vi "Command Move Direction Field (Gyro Hold).vi"(2 "Input Robot System Funtions":T1, 3 "Cmd Parameter 1":dbl, 4 "Cmd Parameter 2":dbl, 5 "Startup":bool) -> (0 "Output Robot System Functions":T1, 1 "Completed":bool)   [LabVIEW 2014]
uses:
  Subsystems VIs/Robot Commands.ctl
  Command Execution State.ctl
  Global Variables/Sensor Data (Edited).vi
  Global Variables/Settings.vi
panel:
  out "PID Tracking":cluster{"Goal Wheel Position":dbl, dbl}(graph)={"Goal Wheel Position"=0.0, -90.17571233858979}
  # "Sample robot\ncontrol output.\nReplace with \nactual teleop \ncontrol signal \nstructure."
  # "Field Centric"
  # "Field Centric"
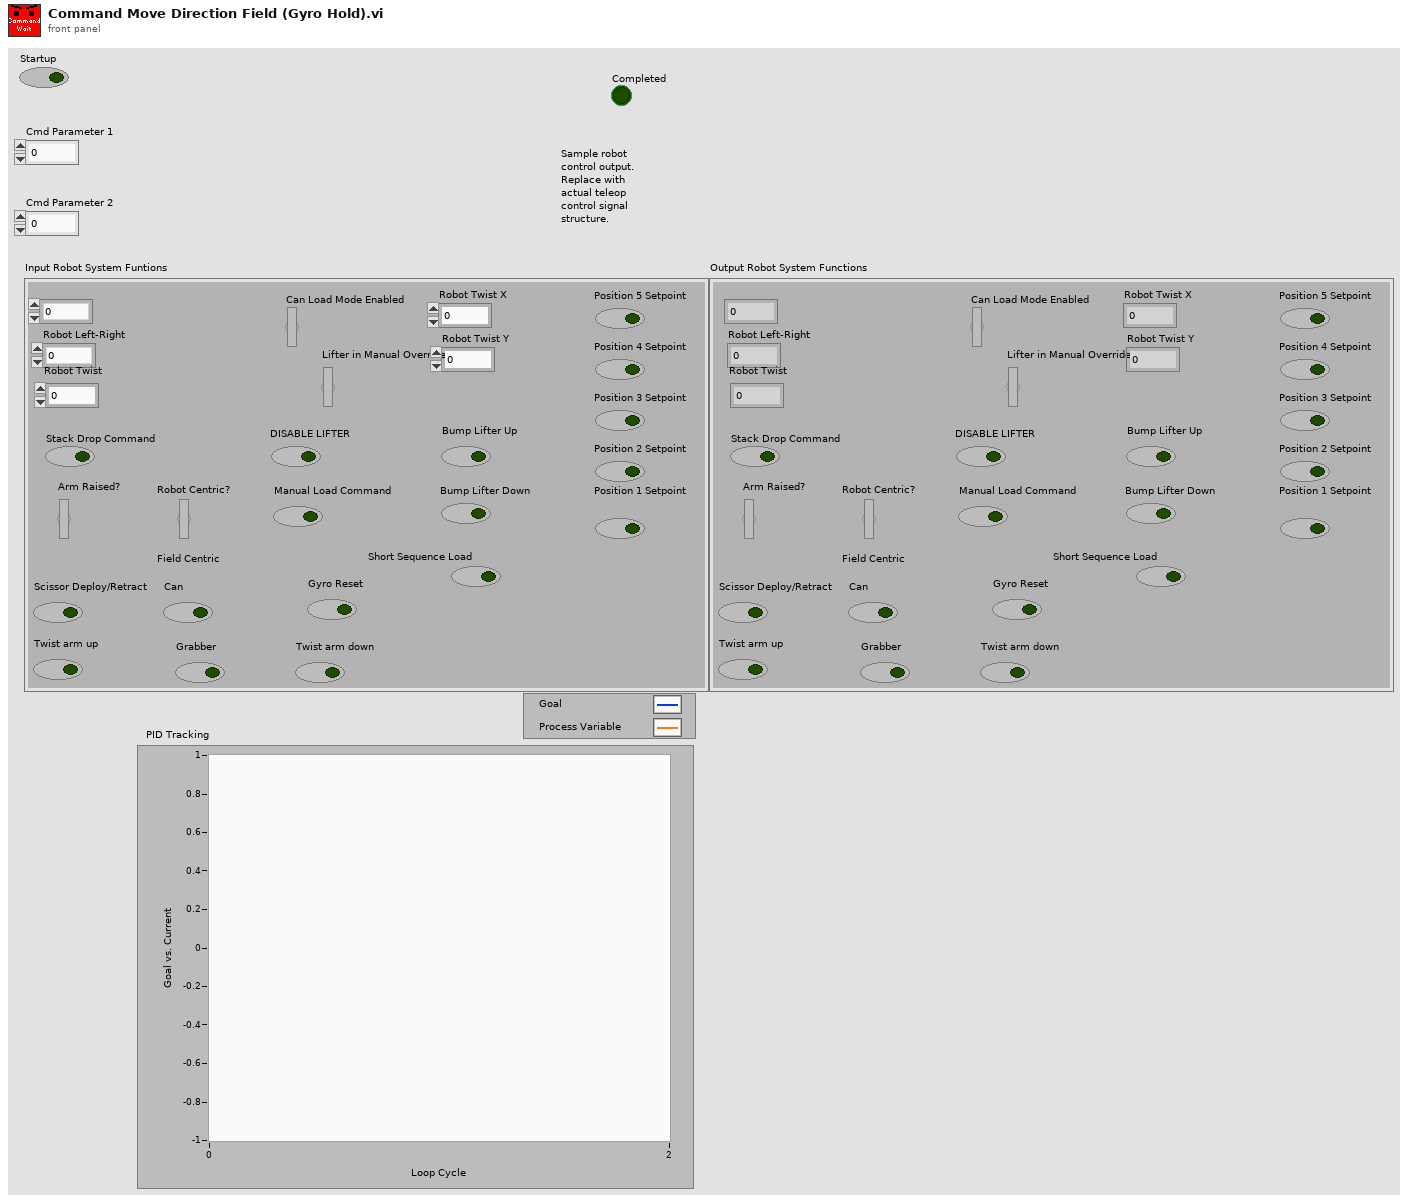
[diagram p1: front panel]
types:
  T1 = typedef "Robot Commands.ctl" = cluster{"Robot Forward-Reverse":dbl, "Robot Left-Right":dbl, "Robot Twist":dbl, "Can Load Mode Enabled":bool, "Lifter in Manual Override?":bool, "Stack Drop Command":bool, "Arm Raised?":bool, "DISABLE LIFTER":bool, "Position 1 Setpoint":bool, "Position 2 Setpoint":bool, "Position 3 Setpoint":bool, "Position 4 Setpoint":bool, "Position 5 Setpoint":bool, "Bump Lifter Down":bool, "Bump Lifter Up":bool, "Manual Load Command":bool, "Robot Centric?":bool, "Scissor Deploy/Retract":bool, "Grabber":bool, "Can":bool, "Twist arm up":bool, "Gyro Reset":bool, "Twist arm down":bool, "Short Sequence Load":bool, "Robot Twist X":dbl, "Robot Twist Y":dbl}
  T2 = typedef "Command Execution State.ctl" = enum16{"Initialize", "Execute", "Finish"}
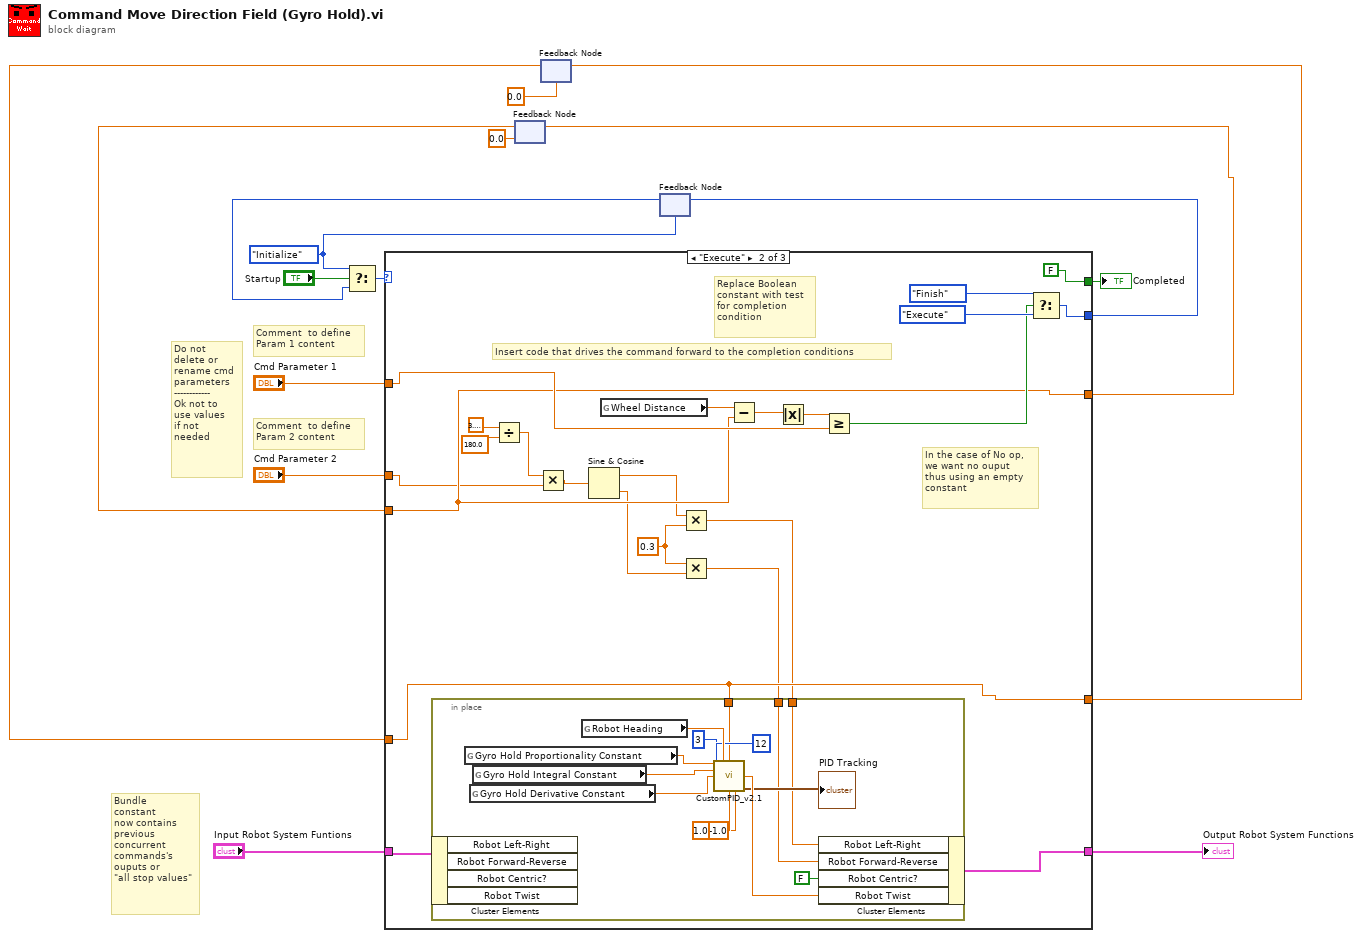
[diagram p0: block diagram]
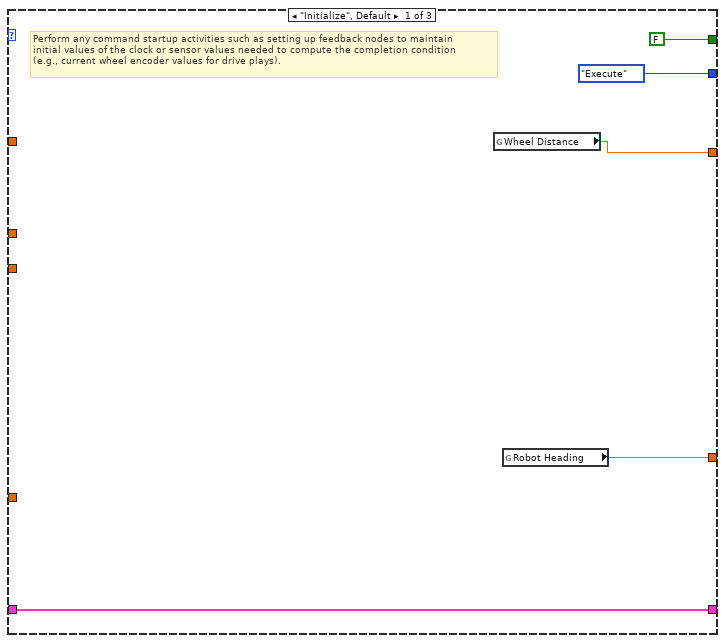
[diagram p2: hidden frame]
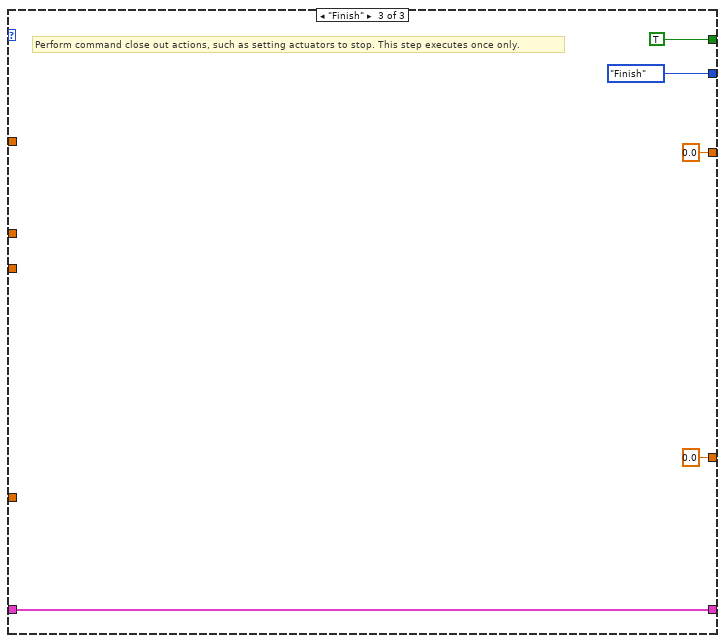
[diagram p3: hidden frame]
diagram:
  w11 = Command_Execution_State."Initialize" ("Play State")
  # "Bundle \nconstant\nnow contains\nprevious \nconcurrent\ncommands's\nouputs or\n\"all stop values\""
  # "Do not \ndelete or\nrename cmd\nparameters\n------------\nOk not to \nuse values\nif not \nneeded"
  # "Comment  to define\nParam 2 content"
  # "Comment  to define\nParam 1 content"
  n1 = feedback #1(0.0 ("Wheel Distance")) -> (w5:dbl)
  n2 = feedback #2(0.0 ("Wheel Distance")) -> (w2:dbl)
  n3 = feedback #3(w11) -> (w12:T2)
  n4 = Select(t=w11, s="Startup", f=w12) -> (s? t:f=w16:T2)
  n5 = case shown="\"Execute\"" w16 {
    tunnel: [FALSE FALSE TRUE] -> w14
    tunnel: [Command_Execution_State."Execute" ("Play State") w35 Command_Execution_State."Finish" ("f")] -> w13
    tunnel: "Cmd Parameter 1" -> [_ w36 _]
    tunnel: "Cmd Parameter 2" -> [_ w29 _]
    tunnel: [w19 w37 w59] -> w7
    tunnel: "Input Robot System Funtions" -> [w19 w38 w59]
    tunnel: [w18 w33 0.0 ("Wheel Distance")] -> w6
    tunnel: w5 -> [_ w33 _]
    tunnel: [w17 w28 0.0 ("Wheel Distance")] -> w3
    tunnel: w2 -> [_ w28 _]
    frame "Initialize", Default {
      # "Perform any command startup activities such as setting up feedback nodes to maintain \ninitial values of the clock or sensor values needed to compute the completion condition\n(e.g., current wheel encoder values for drive plays)."
      n6 = global read "Sensor Data (Edited).vi" "Wheel Distance"() -> (w18:dbl)
      n7 = global read "Sensor Data (Edited).vi" "Robot Heading"() -> (w17:dbl)
    }
    frame "Execute" {
      w24 = 0.3
      # "In the case of No op, \nwe want no ouput \nthus using an empty \nconstant"
      # "Replace Boolean\nconstant with test \nfor completion \ncondition"
      # "Insert code that drives the command forward to the completion conditions"
      n8 = Divide(x=3.141592653589793, y=180.0) -> (x/y=w30:dbl)
      n9 = Multiply(x=w30, y=w29) -> (x*y=w27:dbl)
      n10 = Sine & Cosine(0:w27) -> (1:w26:dbl, 2:w25:dbl)
      n11 = global read "Sensor Data (Edited).vi" "Wheel Distance"() -> (w44:dbl)
      n12 = Multiply(x=w26, y=w24) -> (x*y=w22:dbl)
      n13 = Multiply(x=w24, y=w25) -> (x*y=w23:dbl)
      n14 = in-place {
        in-place-border: w28 -> [w47]
        in-place-border: w23 -> [w45]
        in-place-border: w22 -> [w46]
        n15 = in-place-cluster #4(w38) -> ()  [unwired: 4 out]
        n16 = global read "Settings.vi" "Gyro Hold Proportionality Constant"() -> (w51:dbl)
        n17 = global read "Settings.vi" "Gyro Hold Derivative Constant"() -> (w49:dbl)
        n18 = global read "Settings.vi" "Gyro Hold Integral Constant"() -> (w50:dbl)
        n19 = global read "Sensor Data (Edited).vi" "Robot Heading"() -> (w56:dbl)
        n20 = call "CustomPID_v2.1.vi"("Kp"=w51, "Process Variable"=w56, "Goal"=w47, "Ki"=w50, "Kd"=w49, "N-Diff"=3, "N-Int"=12, "Max Ouput"=1.0, "Min Output"=-1.0) -> ("Command"=w57:dbl, "PID Tracking"=→"PID Tracking":cluster{"Goal Wheel Position":dbl, dbl})  [unwired: 4 in, 1 out]
        n21 = in-place-cluster #4("Robot Left-Right"=w46, "Robot Forward-Reverse"=w45, "Robot Centric?"=FALSE, "Robot Twist"=w57) -> (w37:T1)
      }
      n22 = Subtract(x=w44, y=w33) -> (x-y=w40:dbl)
      n23 = Absolute Value(x=w40) -> (abs(x)=w39:dbl)
      n24 = Greater Or Equal?(x=w39, y=w36) -> (x >= y?=w42:bool)
      n25 = Select(t=Command_Execution_State."Finish" ("Play State"), s=w42, f=Command_Execution_State."Execute" ("Play State")) -> (s? t:f=w35:T2)
    }
    frame "Finish" {
      # "Perform command close out actions, such as setting actuators to stop. This step executes once only."
    }
  }
  "Completed" <- w14
  "Output Robot System Functions" <- w7
  n26 = feedback-in #1(w6) -> ()
  n27 = feedback-in #2(w3) -> ()
  n28 = feedback-in #3(w13) -> ()
